vi "Save module.vi"(7 "Acquisition mode":T1, 8 "error in":errorcluster, 9 "path":path=path "C:/Users/BOAS-USER/Documents/Data/0520/test", 10 "#A lines":i32=1250, 11 "#B lines":i32) -> (0 "error out":errorcluster)   [LabVIEW 2018]
uses:
  type defines/FFT mode.ctl
  Controls/Queue Manager Actions.ctl
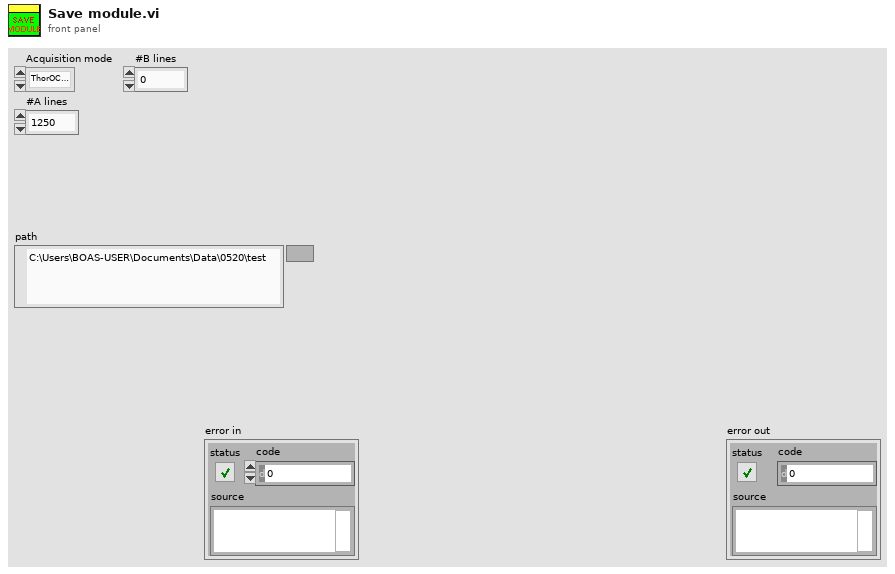
[diagram p1: front panel]
types:
  T1 = typedef "FFT mode.ctl" = enum16{"ThorOCT B line", "ThorOCT Spectral", "ThorOCT FFT", "Alazar B line", "Alazar FFT", "GPU FFT", "Alazar Spectral"}
  T2 = typedef "Queue Manager Actions.ctl" = enum16{"Init", "Enqueue", "Enqueue All", "Preview Queue", "Dequeue", "Get Status", "Flush Queue", "Flush All Queues", "Release All Queues", "Release Queue", "Enqueue at Opposite End"}
  T3 = enum16{"open", "replace", "create", "open or create", "replace or create", "replace or create with confirmation"}
  T4 = enum16{"big-endian, network order", "native, host order", "little-endian"}
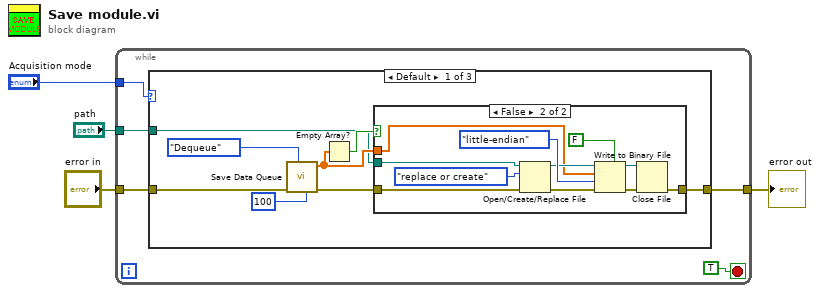
[diagram p0: block diagram]
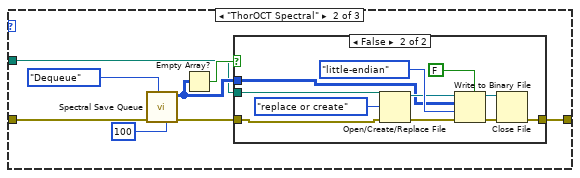
[diagram p3: hidden frame]
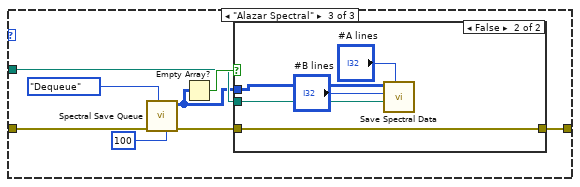
[diagram p5: hidden frame]
diagram:
  n1 = while {
    tunnel: "error in" -> [w9]
    tunnel: "path" -> [w6]
    tunnel: "Acquisition mode" -> [w7]
    tunnel: [w5] -> w1
    stop <- TRUE stop-if-true
    n2 = case shown="Default" w7 {
      tunnel: w9 -> [w17 w37 w57]
      tunnel: w6 -> [w11 w30 w51]
      tunnel: [w10 w31 w52] -> w5
      frame Default {
        n3 = call "Save Data Queue.vi"("timeout in ms (-1)"=100, "Action"=Queue_Manager_Actions."Dequeue", "error in (no error)"=w17) -> ("error out"=w13:errorcluster, "data out"=w12:sgl[])  [unwired: 5 in, 2 out]
        n4 = Empty Array?(array=w12) -> (empty?=w14:bool)
        n5 = case shown="False" w14 {
          tunnel: w13 -> [w18 w26]
          tunnel: w12 -> [_ w20]
          tunnel: [w18 w23] -> w10
          tunnel: w11 -> [_ w19]
          frame True {
          }
          frame False {
            n6 = Open/Create/Replace File(file path (use dialog)=w19, error in=w26, operation (0:open)=T3."replace or create") -> (refnum out=w22:refnum<file>, error out=w25:errorcluster)  [unwired: 3 in, 1 out]
            n7 = Write to Binary File(file (use dialog)=w22, data=w20, error in=w25, 5:FALSE ("prepend array or string size? (T)"), 9:T4."little-endian" ("byte order (0:big-endian, network order)")) -> (refnum out=w21:refnum<file>, error out=w24:errorcluster)  [unwired: 1 in, 1 out]
            n8 = Close File(refnum=w21, error in=w24) -> (error out=w23:errorcluster)  [unwired: 1 out]
          }
        }
      }
      frame "ThorOCT Spectral" {
        n9 = call "Spectral Save Queue.vi"("timeout in ms (-1)"=100, "Action"=Queue_Manager_Actions."Dequeue", "error in (no error)"=w37) -> ("error out"=w34:errorcluster, "data out"=w32:u16[][])  [unwired: 5 in, 2 out]
        n10 = Empty Array?(array=w32) -> (empty?=w33:bool)
        n11 = case shown="False" w33 {
          tunnel: w34 -> [w38 w46]
          tunnel: [w38 w43] -> w31
          tunnel: w32 -> [_ w40]
          tunnel: w30 -> [_ w39]
          frame True {
          }
          frame False {
            n12 = Open/Create/Replace File(file path (use dialog)=w39, error in=w46, operation (0:open)=T3."replace or create") -> (refnum out=w42:refnum<file>, error out=w45:errorcluster)  [unwired: 3 in, 1 out]
            n13 = Write to Binary File(file (use dialog)=w42, data=w40, error in=w45, 5:FALSE ("prepend array or string size? (T)"), 9:T4."little-endian" ("byte order (0:big-endian, network order)")) -> (refnum out=w41:refnum<file>, error out=w44:errorcluster)  [unwired: 1 in, 1 out]
            n14 = Close File(refnum=w41, error in=w44) -> (error out=w43:errorcluster)  [unwired: 1 out]
          }
        }
      }
      frame "Alazar Spectral" {
        n15 = call "Spectral Save Queue.vi"("timeout in ms (-1)"=100, "Action"=Queue_Manager_Actions."Dequeue", "error in (no error)"=w57) -> ("error out"=w54:errorcluster, "data out"=w50:u16[][])  [unwired: 5 in, 2 out]
        n16 = Empty Array?(array=w50) -> (empty?=w53:bool)
        n17 = case shown="False" w53 {
          tunnel: w54 -> [w58 w59]
          tunnel: [w58 w59] -> w52
          tunnel: w50 -> [_ w63]
          tunnel: w51 -> [_ w62]
          frame True {
          }
          frame False {
            n18 = call "Save Spectral Data.vi"("#A lines"="#A lines", "file path"=w62, "#B lines"="#B lines", "data in"=w63) -> ()  [unwired: 8 in]
          }
        }
      }
    }
  }
  "error out" <- w1
